vi "fil ter matrix.vi"(7 "matrix":dbl[](array[numeric])=array[4097 elements], 9 "multiplication/ substitution":i16(ring) items=["subst", "mult"], 10 "intensity / phase":i16(ring) items=["int", "pha"], 11 "field":T1) -> (3 "field out":T1, 5 "matrix out":dbl[](array[numeric]))   [LabVIEW 2012, in "Lightpipes.lvlib"]
doc: "__declspec(dllexport) void fil_ter_matrix(FIELD* field, const char* c1, const char* c2, double matrix[]);"
uses:
  LightPipes.lvlib
  VS Project/Debug/Lightpipes.dll
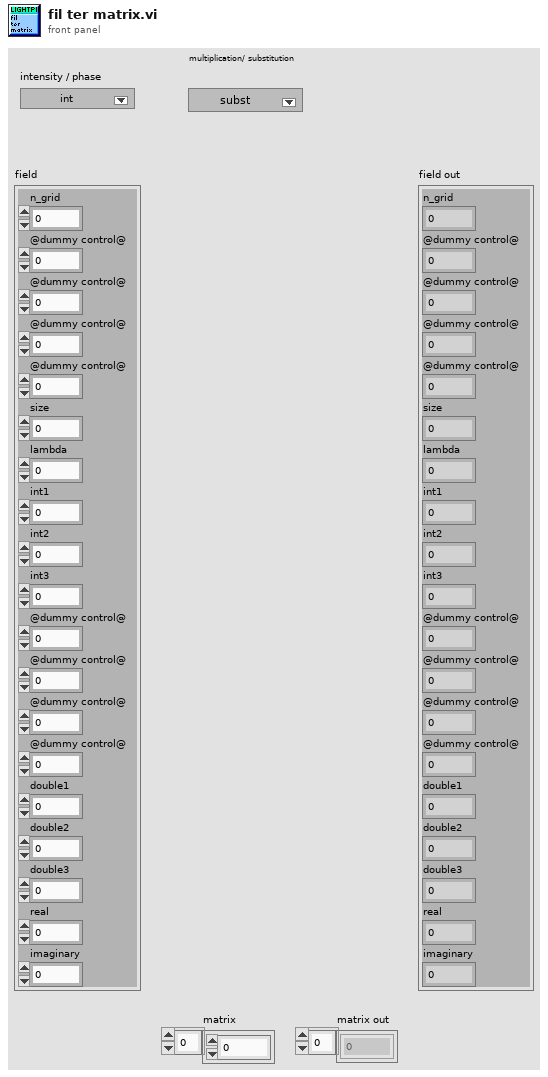
[diagram p1: front panel]
types:
  T1 = cluster{"n_grid":i32, "@dummy control@":i8, "@dummy control@":i8, "@dummy control@":i8, "@dummy control@":i8, "size":dbl, "lambda":dbl, "int1":i32, "int2":i32, "int3":i32, "@dummy control@":i8, "@dummy control@":i8, "@dummy control@":i8, "@dummy control@":i8, "double1":dbl, "double2":dbl, "double3":dbl, "real":u32, "imaginary":u32}
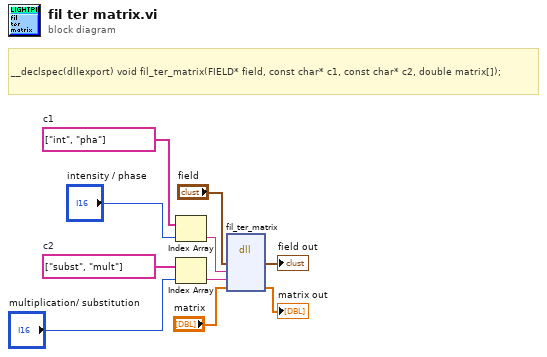
[diagram p0: block diagram]
diagram:
  w4 = string[] ["int", "pha"]  # c1
  w6 = string[] ["subst", "mult"]  # c2
  # "__declspec(dllexport) void fil_ter_matrix(FIELD* field, const char* c1, const char* c2, double matrix[]);"
  n1 = Index Array(array=w4, index="intensity / phase") -> (element=w2:string)
  n2 = Index Array(array=w6, index="multiplication/ substitution") -> (element=w1:string)
  n3 = dll-call lib="C:/Users/Tri/Documents/Lightpipes/VS Project/Debug/Lightpipes.*" fn="fil_ter_matrix"("field"="field", "c1"=w2, "c2"=w1, "matrix"="matrix") -> ("field"=→"field out":T1, "matrix"=→"matrix out":dbl[])  [unwired: 6 in, 2 out]
